vi "Handle Last Ack Core.vi"(4 "error in":errorcluster, 6 "Last Ack":refnum<class "Last Ack.lvclass">, 7 "CRIO MSS Test Actor in":refnum<class "CRIO MSS Test Actor.lvclass">) -> (0 "error out":errorcluster, 3 "CRIO MSS Test Actor out":refnum<class "CRIO MSS Test Actor.lvclass">)   [LabVIEW 2023, in "CRIO MSS Test Actor.lvlib" / "CRIO MSS Test Actor.lvclass"]
doc: "(<B>Filename</B>: Actor Framework.lvlib:Actor.lvclass:Handle Last Ack Core.vi)\n\nDefines how the caller actor responds to the Last Ack message from a nested actor. The Last Ack message is the final message a nested actor sends to its caller before it shuts down. The message contains information about the final state of the nested actor.\n\nBy default, this method does nothing except return any error the nested actor sent. A descendant class may override this method to define behavior."
uses:
  CRIO MSS Test Actor.lvclass
  CRIO MSS Test Actor.lvclass/CRIO MSS Test Actor.ctl
  <vilib>/ActorFramework/Actor/Actor.lvclass
  <vilib>/ActorFramework/LastAck/Last Ack.lvclass
  C:/Program Files/National Instruments/LabVIEW 2023/vi.lib/ActorFramework/Actor/Actor.lvclass
  D:/git/HAL/HAL GOOP4/Host Measure and Stimulus Subsystems/Tests/CRIO MSS Test Actor/CRIO MSS Test Actor/CRIO MSS Test Actor.lvclass
  D:/git/HAL/HAL GOOP4/Host Measure and Stimulus Subsystems/Tests/CRIO MSS Test Actor/ICRIO MSS Test Actor/ICRIO MSS Test Actor.lvclass
  C:/Program Files/National Instruments/LabVIEW 2023/vi.lib/ni/Actors/Network Endpoint Actors/Nested Endpoint Caller/Nested Endpoint Caller/Nested Endpoint Caller.lvclass
  <vilib>/ActorFramework/Message Enqueuer/Message Enqueuer.lvclass
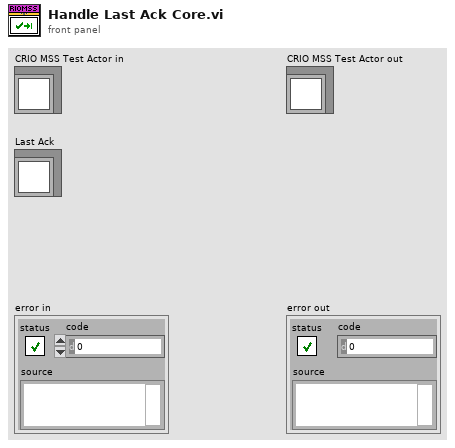
[diagram p1: front panel]
types:
  T1 = map{string, refnum<class "Message Enqueuer.lvclass">}
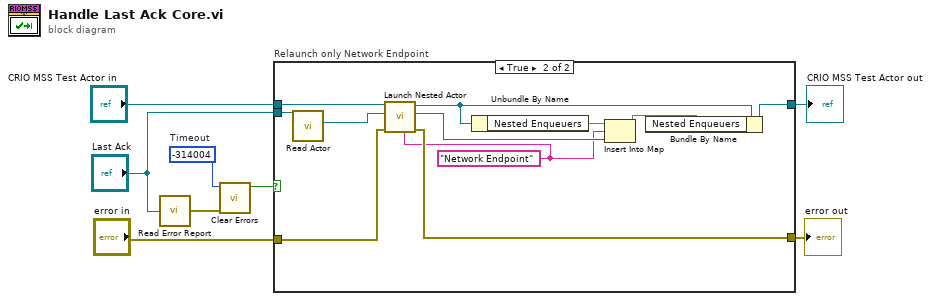
[diagram p0: block diagram]
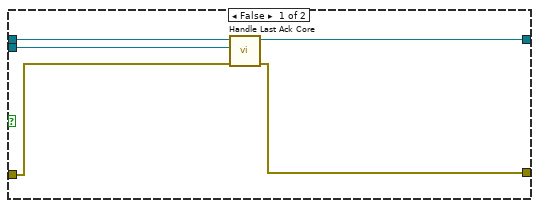
[diagram p2: hidden frame]
diagram:
  w7 = -314004  # Timeout
  n1 = call <vilib>:"Read Error Report.vi"("Last Ack"="Last Ack") -> ("error report"=w8:errorcluster)
  n2 = call <vilib>:"Clear Errors.vi"("error in (no error)"=w8, "specific error code to clear (0: all)"=w7) -> ("specific error cleared?"=w6:bool)  [unwired: 4 in, 1 out]
  n3 = case "Relaunch only Network Endpoint" shown="True" w6 {
    tunnel: "CRIO MSS Test Actor in" -> [w13 w24]
    tunnel: [w11 w23] -> w4
    tunnel: [w12 w19] -> w5
    tunnel: "Last Ack" -> [w10 w16]
    tunnel: "error in" -> [w9 w14]
    frame False {
      n4 = call-parent "Handle Last Ack Core.vi"("error in (no error)"=w9, "Last Ack"=w10, "Actor in"=w13) -> ("error out"=w11:errorcluster, "Actor out"=w12:refnum<class "CRIO MSS Test Actor.lvclass">)  [unwired: 3 in]
    }
    frame True {
      w17 = "Network Endpoint" ("key")
      n5 = call <vilib>:"Read Actor.vi"("Last Ack"=w16) -> ("Actor"=w15:refnum<class "Actor.lvclass">)  [unwired: 10 in]
      n6 = call <vilib>:"Launch Nested Actor.vi"("Debug Alias"=w17, "error in (no error)"=w14, "Nested Actor"=w15, "Caller Actor in"=w24) -> ("error out"=w23:errorcluster, "Nested Actor's Enqueuer"=w20:refnum<class "Message Enqueuer.lvclass">, "Caller Actor out"=w22:refnum<class "CRIO MSS Test Actor.lvclass">)  [unwired: 5 in]
      n7 = Unbundle By Name(w22) -> ("Nested Enqueuers"=w21)
      n8 = Insert Into Map(map in=w21, key=w17, value=w20) -> (map out=w18:T1)  [unwired: 2 out]
      n9 = Bundle By Name(cluster=w22, "Nested Enqueuers"=w18) -> (w19:refnum<class "CRIO MSS Test Actor.lvclass">)
    }
  }
  "CRIO MSS Test Actor out" <- w5
  "error out" <- w4
